vi "optogeneticsGetCoordsFromReferences.vi"(0 "index":u16, 1 "sizex2":u16=256, 2 "hamamatsuFrameAvailableReferences":refnum<data-value>[](array[refnum]), 3 "hamamatsuFrameReferences":refnum<data-value>[](array[refnum]), 5 "segmentationNeuronXYLatestVolume":refnum<data-value>[](array[refnum]), 7 "segmentationNeuronNLatestVolume":refnum<data-value>[](array[refnum]), 9 "segmentationZLatestVolume":refnum<data-value>[](array[refnum]), 11 "segmentationFrameCountLatestVolume":refnum<data-value>[](array[refnum]), 13 "wait":bool=TRUE) -> (4 "x":u16, 6 "y":u16, 8 "z":u16, 10 "z (true vals)":dbl[](array[numeric]), 15 "frame count":i32)   [LabVIEW 2017]
uses:
  globalUtilities.vi
panel:
  out "Waveform Graph":u16[](graph)
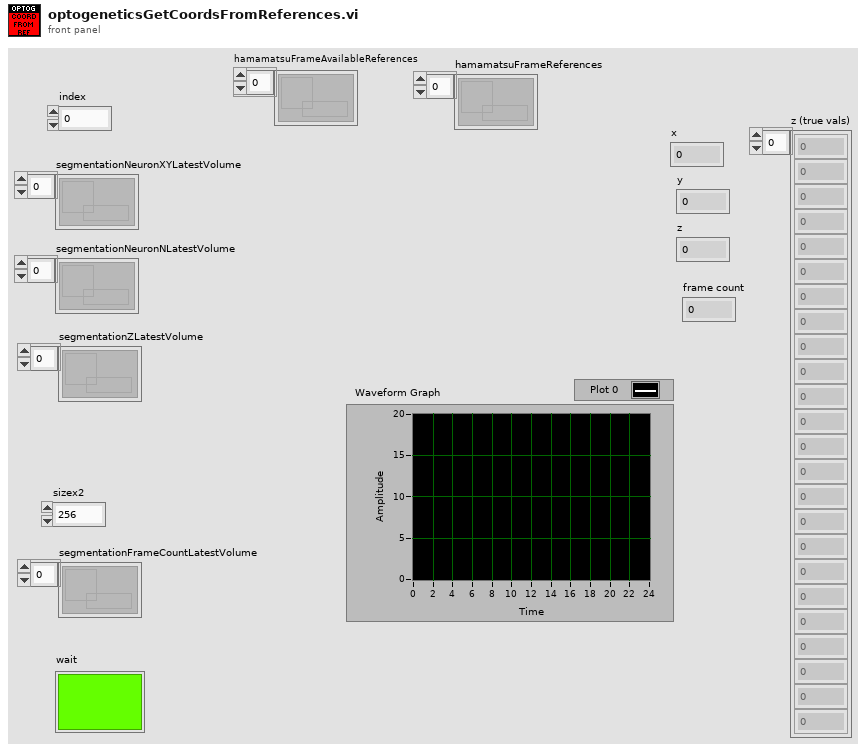
[diagram p1: front panel]
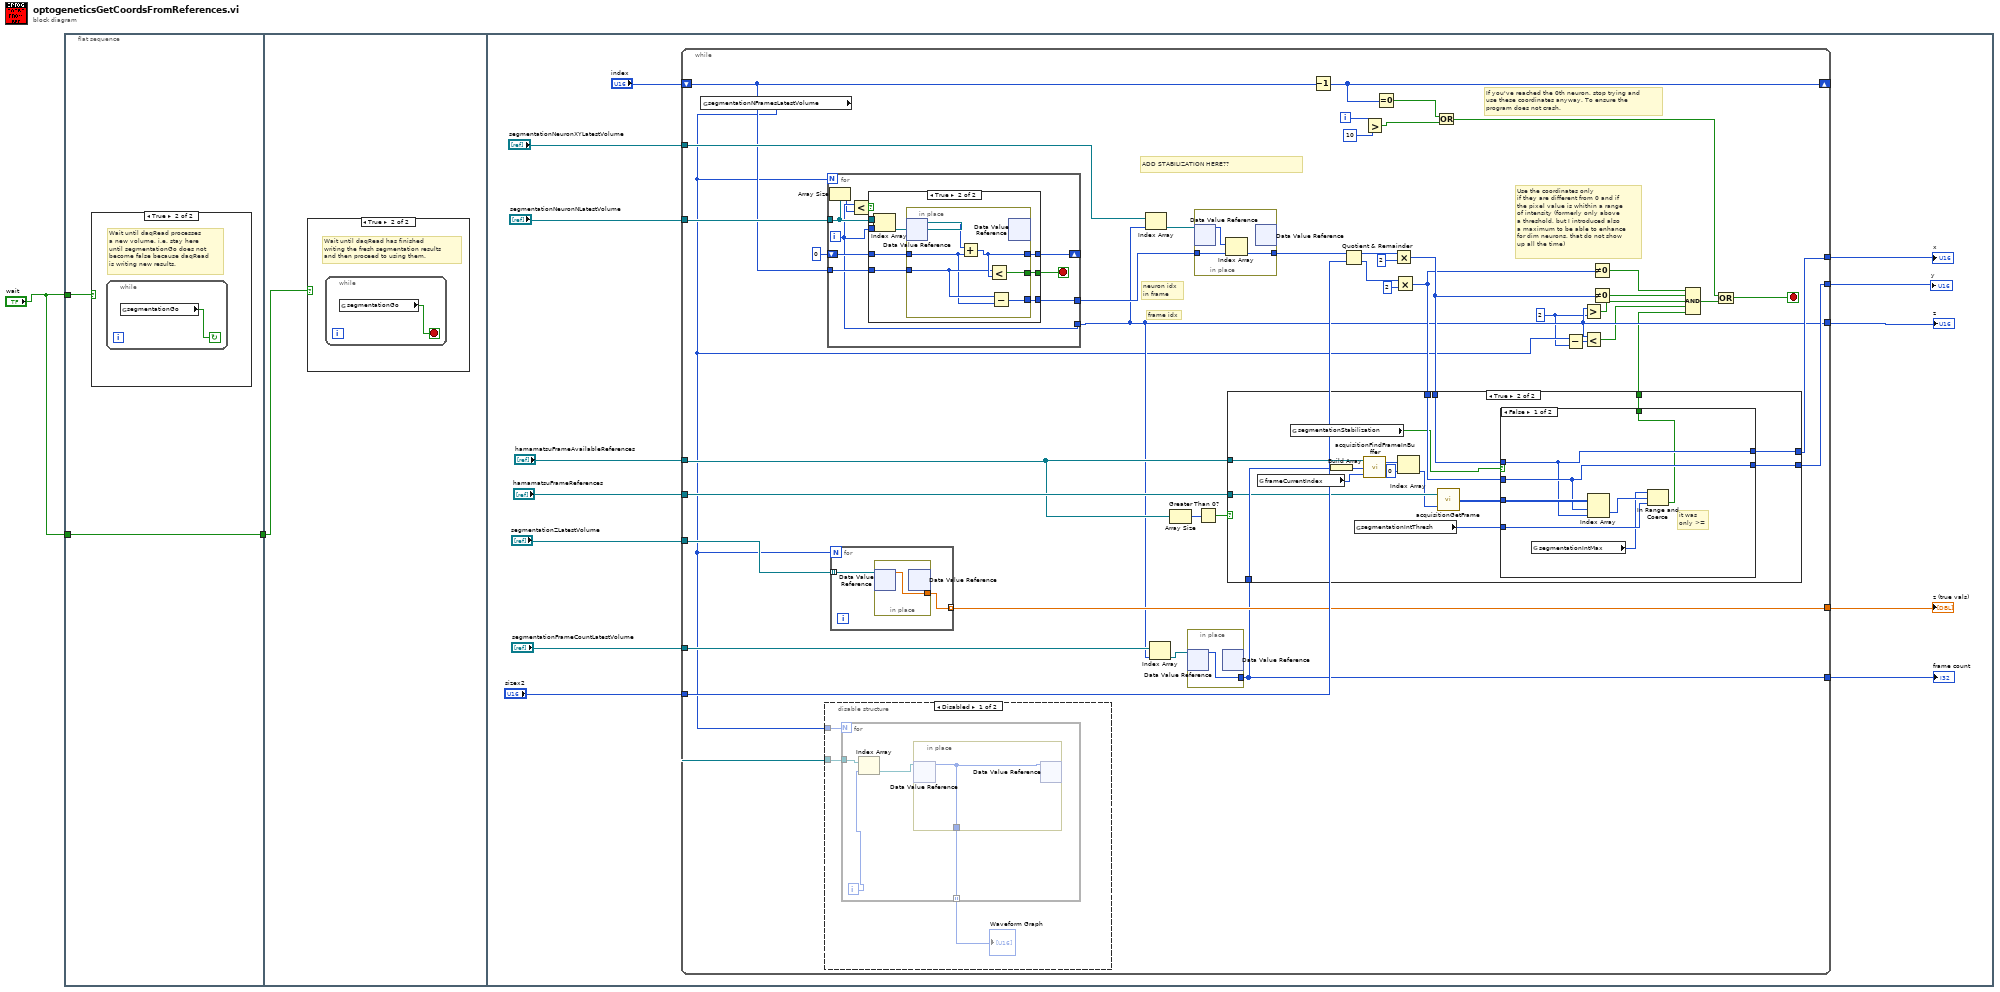
[diagram p0: block diagram]
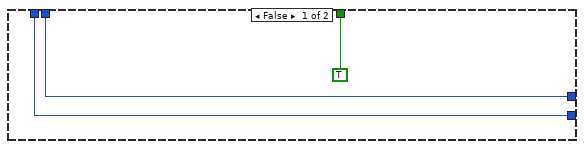
[diagram p4: hidden frame]
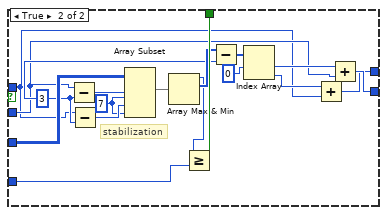
[diagram p5: hidden frame]
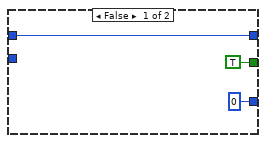
[diagram p7: hidden frame]
diagram:
  n1 = flat-sequence {
    tunnel: "wait" -> [w4]
    tunnel: [w3] -> w2
    tunnel: "wait" -> [w3]
    tunnel: w2 -> [w6]
    frame #0 {
      n2 = case shown="True" w4 {
        frame False {
        }
        frame True {
          # "Wait until daqRead processes\na new volume, i.e. stay here\nuntil segmentationGo does not\nbecome false because daqRead \nis writing new results."
          n3 = while {
            stop <- w5 continue-if-true
            n4 = global read "globalUtilities.vi" "segmentationGo"() -> (w5:bool)
          }
        }
      }
    }
    frame #1 {
      n5 = case shown="True" w6 {
        frame False {
        }
        frame True {
          # "Wait until daqRead has finished\nwriting the fresh segmentation results\nand then proceed to using them."
          n6 = while {
            stop <- w7 stop-if-true
            n7 = global read "globalUtilities.vi" "segmentationGo"() -> (w7:bool)
          }
        }
      }
    }
    frame #2 {
      n8 = while {
        tunnel: "segmentationNeuronXYLatestVolume" -> [w61]
        tunnel: "sizex2" -> [w53]
        tunnel: "segmentationZLatestVolume" -> [w52]
        tunnel: [w51] -> w16
        tunnel: "segmentationNeuronNLatestVolume" -> [w50]
        tunnel: "segmentationFrameCountLatestVolume" -> [w49]
        tunnel: "hamamatsuFrameAvailableReferences" -> [w37]
        tunnel: [w47] -> w11
        tunnel: "hamamatsuFrameReferences" -> [w46]
        tunnel: [w34] -> w9
        tunnel: [w33] -> w8
        tunnel: [w26] -> w13
        shift-right: [w42] -> _
        shift-left: "index" -> [w43]
        i -> [w32]
        stop <- w41 stop-if-true
        w24 = 2 ("y")
        # "Use the coordinates only\nif they are different from 0 and if\nthe pixel value is whithin a range\nof intensity (formerly only above\na threshold, but I introduced also\na maximum to be able to enhance\nfor dim neurons, that do not show\nup all the time)"
        # "If you've reached the 0th neuron, stop trying and\nuse these coordinates anyway. To ensure the \nprogram does not crash."
        # "neuron idx\nin frame"
        # "frame idx"
        # "ADD STABILIZATION HERE??"
        n9 = global read "globalUtilities.vi" "segmentationNFramesLatestVolume"() -> (w25:i32)
        n10 = disable-structure shown="Disabled" {
          disable-tunnel: w25 -> [w110 _]
          disable-tunnel: w50 -> [w109 _]
          frame Disabled {
            n11 = for {
              N: w110 -> [_]
              tunnel: w109 -> [w114]
              tunnel: [w112] -> w108 mode=indexing
              i -> [w111]
              n12 = Index Array(array=w114, index=w111) -> (element=w113:refnum<data-value>)
              n13 = in-place {
                in-place-border: [w115] -> w112
                n14 = in-place-dvr #1(w113) -> (w115:u16)  [unwired: 1 out]
                n15 = in-place-dvr #1(w115) -> ()  [unwired: 2 out]
              }
            }
            "Waveform Graph" <- w108
          }
          frame Enabled {
          }
        }
        n16 = for {
          N: w25 -> [_]
          tunnel: w50 -> [w125]
          shift-right: [w129] -> _
          shift-left: u16 0 -> [w130]
          tunnel: w43 -> [w128]
          tunnel: [w126] -> w59
          tunnel: [w124] -> w26
          i -> [w124]
          stop <- w127 stop-if-true
          n17 = Array Size(array=w125) -> (size(s)=w122:i32)
          n18 = Less?(x=w124, y=w122) -> (x < y?=w123:bool)
          n19 = case shown="True" w123 {
            tunnel: w130 -> [w133 w140]
            tunnel: [w133 w139] -> w129
            tunnel: w128 -> [_ w138]
            tunnel: [TRUE w137] -> w127
            tunnel: [u16 0 w136] -> w126
            tunnel: w124 -> [_ w135]
            tunnel: w125 -> [_ w134]
            frame False {
            }
            frame True {
              n20 = Index Array(array=w134, index=w135) -> (element=w141:refnum<data-value>)
              n21 = in-place {
                in-place-border: w140 -> [w143]
                in-place-border: [w146] -> w139
                in-place-border: w138 -> [w144]
                in-place-border: [w145] -> w137
                in-place-border: [w142] -> w136
                n22 = in-place-dvr #2(w141) -> (w147:u16)  [unwired: 1 out]
                n23 = Add(x=w147, y=w143) -> (x+y=w146:u16)
                n24 = Less?(x=w144, y=w146) -> (x < y?=w145:bool)
                n25 = Subtract(x=w144, y=w143) -> (x-y=w142:u16)
                n26 = in-place-dvr #2() -> ()  [unwired: 1 in, 2 out]
              }
            }
          }
        }
        n27 = for {
          N: w25 -> [_]
          tunnel: w52 -> [w117] mode=indexing
          tunnel: [w116] -> w51 mode=indexing
          n28 = in-place {
            in-place-border: [w118] -> w116
            n29 = in-place-dvr #3(w117) -> (w118:dbl)  [unwired: 1 out]
            n30 = in-place-dvr #3() -> ()  [unwired: 1 in, 2 out]
          }
        }
        n31 = Index Array(array=w61, index=w26) -> (element=w60:refnum<data-value>)
        n32 = Index Array(array=w49, index=w26) -> (element=w48:refnum<data-value>)
        n33 = Array Size(array=w37) -> (size(s)=w35:i32)
        n34 = in-place {
          in-place-border: [w107] -> w47
          n35 = in-place-dvr #4(w48) -> (w107:i32)  [unwired: 1 out]
          n36 = in-place-dvr #4() -> ()  [unwired: 1 in, 2 out]
        }
        n37 = in-place {
          in-place-border: w59 -> [w120]
          in-place-border: [w119] -> w54
          n38 = in-place-dvr #5(w60) -> (w121:u16[])  [unwired: 1 out]
          n39 = Index Array(array=w121, index=w120) -> (element=w119:u16)
          n40 = in-place-dvr #5() -> ()  [unwired: 1 in, 2 out]
        }
        n41 = Greater Than 0?(x=w35) -> (x > 0?=w36:bool)
        n42 = Decrement(x=w43) -> (x-1=w42:u16)
        n43 = Quotient & Remainder(x=w54, y=w53) -> (x-y*floor(x/y)=w57:u16, floor(x/y)=w58:u16)
        n44 = Greater?(x=w32, y=10) -> (0:w30:bool)
        n45 = Equal To 0?(x=w42) -> (x = 0?=w29:bool)
        n46 = Multiply(x=w57, y=u16 2) -> (x*y=w45:u16)
        n47 = Multiply(x=w58, y=u16 2) -> (x*y=w44:u16)
        n48 = case shown="True" w36 {
          tunnel: w37 -> [_ w81]
          tunnel: w47 -> [_ w80]
          tunnel: w46 -> [_ w75]
          tunnel: w45 -> [w64 w67]
          tunnel: w44 -> [w63 w68]
          tunnel: [TRUE w72] -> w22
          tunnel: [w64 w69] -> w34
          tunnel: [w63 w70] -> w33
          frame False {
          }
          frame True {
            n49 = global read "globalUtilities.vi" "frameCurrentIndex"() -> (w78:i32)
            n50 = global read "globalUtilities.vi" "segmentationStabilization"() -> (w66:bool)
            n51 = Build Array(w80) -> (w79:i32[])
            n52 = global read "globalUtilities.vi" "segmentationIntThresh"() -> (w73:u16)
            n53 = call "acquisitionFindFrameInBuffer.vi"("startBufferIndex"=w78, "frameCounts"=w79, "hamamatsuFrameAvailableReferences"=w81) -> ("frameIndices"=w77:i32[])  [unwired: 1 out]
            n54 = Index Array(array=w77, index=0) -> (element=w74:i32)
            n55 = call "acquisitionGetFrame.vi"("index"=w74, "hamamatsuFrameReferences"=w75) -> ("frameOut"=w71:u16[][])
            n56 = case shown="False" w66 {
              tunnel: w73 -> [w84 w106]
              tunnel: [w82 w105] -> w72
              tunnel: w71 -> [w88 w104]
              tunnel: [w87 w90] -> w70
              tunnel: [w86 w89] -> w69
              tunnel: w68 -> [w87 w92]
              tunnel: w67 -> [w86 w91]
              frame False {
                # "it was\nonly >="
                n57 = global read "globalUtilities.vi" "segmentationIntMax"() -> (w83:u16)
                n58 = Index Array(array=w88, index (row)=w87, index (col)=w86) -> (element=w85:u16)
                n59 = In Range and Coerce(upper limit=w83, x=w85, lower limit=w84) -> (In Range?=w82:bool)  [unwired: 1 out]
              }
              frame True {
                w101 = 7 ("length")
                w99 = u16 3 ("y")
                # "stabilization"
                n60 = Subtract(x=w92, y=w99) -> (x-y=w103:u16)
                n61 = Subtract(x=w91, y=w99) -> (x-y=w102:u16)
                n62 = Array Subset(array=w104, index (row)=w103, length (row)=w101, index (col)=w102, length (col)=w101) -> (w93:u16[][])
                n63 = Array Max & Min(array=w93) -> (max value=w96:u16, max index (indices)=w100:i32[])  [unwired: 2 out]
                n64 = Greater Or Equal?(x=w96, y=w106) -> (x >= y?=w105:bool)
                n65 = Subtract(x=w100, y=w99) -> (x-y=w98:i32[])
                n66 = Index Array(array=w98, index #1=0 ("index")) -> (element #1=w94:i32, element #2=w95:i32)  [unwired: 1 in]
                n67 = Add(x=w95, y=w91) -> (x+y=w89:i32)
                n68 = Add(x=w94, y=w92) -> (x+y=w90:i32)
              }
            }
          }
        }
        n69 = Or(x=w29, y=w30) -> (x .or. y?=w28:bool)
        n70 = Subtract(x=w25, y=w24) -> (x-y=w23:i32)
        n71 = Greater?(x=w26, y=w24) -> (0:w27:bool)
        n72 = Less?(x=w26, y=w23) -> (x < y?=w21:bool)
        n73 = Not Equal To 0?(x=w44) -> (x != 0?=w39:bool)
        n74 = Not Equal To 0?(x=w45) -> (x != 0?=w38:bool)
        n75 = Compound Arithmetic op=AND(w39, w38, w27, w21, w22) -> (w40:bool)
        n76 = Or(x=w28, y=w40) -> (x .or. y?=w41:bool)
      }
      "x" <- w9
      "y" <- w8
      "z" <- w13
      "z (true vals)" <- w16
      "frame count" <- w11
    }
  }
